vi "ReadMultiTof.vi"(8 "error in":errorcluster, 10 "VL6180 Resources":T2[](array[typedef]) {"I2C Slave Address" format="%02x"}, 11 "LINX Resource in":T3) -> (0 "error out":errorcluster, 1 "ToF Readings":T1[](array[typedef]), 2 "VL Configs":T2[](array[typedef]) {"I2C Slave Address" format="%02x"}, 3 "LINX Resoure":T3)   [LabVIEW 2017]
uses:
  Sensors/Time of Flight - VL6180/VL6180 Resource.ctl
  <vilib>/MakerHub/LINX/Private/Type Defs/LINX Ref.ctl
  <vilib>/MakerHub/LINX/Private/Type Defs/Platform.ctl
  <vilib>/MakerHub/LINX/Private/Type Defs/Interface.ctl
  <vilib>/MakerHub/LINX/Private/Device/Type Defs/LINX Device Config.ctl
  <vilib>/MakerHub/LINX/Private/Device/Type Defs/TCP Config.ctl
  <vilib>/MakerHub/LINX/Private/Device/Type Defs/Channels.ctl
  Type Defs/tofReading.ctl
  <vilib>/MakerHub/LINX/LMH-LINX.lvlib
  <vilib>/MakerHub/LINX/Private/Device/Device.lvlib
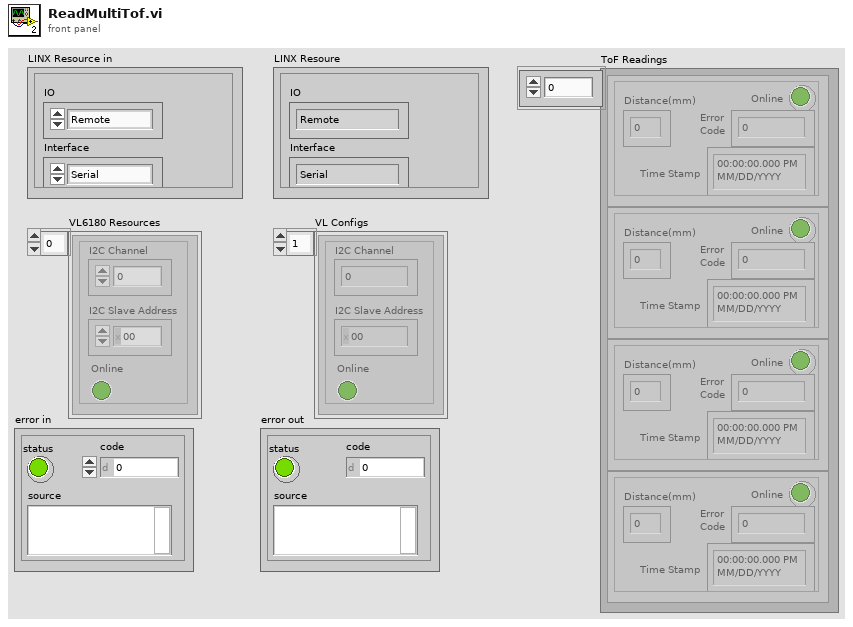
[diagram p1: front panel]
types:
  T1 = typedef "tofReading.ctl" = cluster{"Distance(mm)":u8, "Online":bool, "Error\nCode":u8, "Time Stamp":timestamp}
  T2 = typedef "VL6180 Resource.ctl" = cluster{"I2C Channel":u8, "I2C Slave Address":u8, "Online":bool}
  T3 = typedef "LMH-LINX.lvlib/LINX Ref.ctl" = cluster{"IO":T4, "Interface":T5, "LINX Device Config":T6}
  T4 = typedef "LMH-LINX.lvlib/Platform.ctl" = enum16{"Remote", "Local"}
  T5 = typedef "LMH-LINX.lvlib/Interface.ctl" = enum16{"Serial", "TCP"}
  T6 = typedef "LMH-LINX.lvlib/Device.lvlib/LINX Device Config.ctl" = cluster{"Interface":T5, "COM Port":refnum<visa-resource-name>, "TCP Configuration":T7, "Device Family":u8, "Device ID":u8, "Device Name":string, "TCP Ref":refnum<k5>, "Channels":T8}
  T7 = typedef "LMH-LINX.lvlib/Device.lvlib/TCP Config.ctl" = cluster{"IP Address":string, "Port":u16}
  T8 = typedef "LMH-LINX.lvlib/Channels.ctl" = cluster{"DI":u8[], "DO":u8[], "AI":u8[], "AO":u8[], "PWM":u8[], "QE":u8[], "UART":u8[], "I2C 2":u8[], "SPI":u8[], "CAN":u8[], "Servo":u8[], "AI Ref (V)":dbl, "AI Resolution (Bits)":u8, "AO Ref (V)":dbl, "AO Resolution (Bits)":u8}
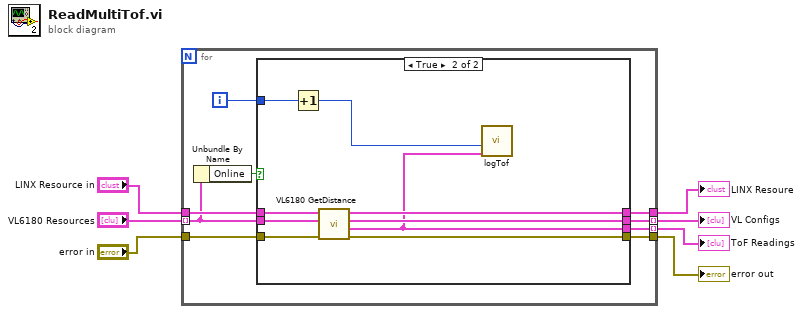
[diagram p0: block diagram]
diagram:
  n1 = for {
    tunnel: "VL6180 Resources" -> [w10] mode=indexing
    tunnel: "LINX Resource in" -> [w16]
    tunnel: "error in" -> [w13]
    tunnel: [w15] -> w6
    tunnel: [w14] -> w7 mode=indexing
    tunnel: [w12] -> w2
    tunnel: [w11] -> w1 mode=indexing
    i -> [w8]
    n2 = Unbundle By Name(w10) -> ("Online"=w9:bool)
    n3 = case shown="True" w9 {
      tunnel: w16 -> [w19 w28]
      tunnel: w10 -> [w18 w27]
      tunnel: [w19 w26] -> w15
      tunnel: [w18 w25] -> w14
      tunnel: w13 -> [w17 w24]
      tunnel: [w17 w23] -> w12
      tunnel: [_ w20] -> w11
      tunnel: w8 -> [_ w22]
      frame False {
      }
      frame True {
        n4 = Increment(x=w22) -> (x+1=w21:i32)
        n5 = call "VL6180 GetDistance.vi"("error in (no error)"=w24, "VL6180 Resource in"=w27, "LINX Resource"=w28) -> ("error out"=w23:errorcluster, "ToF Reading"=w20:T1, "VL6180 Resource out"=w25:T2, "LINX Resource"=w26:T3)  [unwired: 4 in, 1 out]
        n6 = call "logTof.vi"("ToF Reading"=w20, "Index"=w21) -> ()  [unwired: 10 in]
      }
    }
  }
  "error out" <- w2
  "VL Configs" <- w7
  "LINX Resoure" <- w6
  "ToF Readings" <- w1
